vi "ObjDet_Read_Dataset_by_File_Paths_v1.1.vi"(0 "Annotation File Paths":path[](array[path]), 1 "Unique labels":string[](array[string]), 5 "Image File Paths":path[](array[path]), 7 "Img Height":i32, 9 "Img Width":i32, 11 "error in (no error)":errorcluster, 12 "Img Type":enum16{"Grayscale", "RGB"}(ring)) -> (4 "NN_DataSet(In3D_OutBBox)":T1={"Inputs Ref."=variant(refnum<data-value> refnum), "Dataset_Size"=0, "Dims_In"={"C"=0, "H"=0, "W"=0}, "Outputs Refs"=refnum, "No of Classes "=0, "Labels"=[], "File Paths"=[]}, 6 "Anchors":dbl[][](array[numeric]), 8 "Total annotations":i32, 15 "error out":errorcluster)   [LabVIEW 2020]
uses:
  <vilib>/Ngene/Deep Learning Toolkit/Toolkit/NN_Data/API/DataSet/DataSet_Types/NN_DataSet(In3D_OutBBox).ctl
  <vilib>/Ngene/Deep Learning Toolkit/Toolkit/NN_Data/API/NN_Dims(C,H,W).ctl
  <vilib>/Ngene/Deep Learning Toolkit/Toolkit/NN_Data/Controls/DataRef_Types/1D/NN_Data_ref(1D_BBox).ctl
  <vilib>/Ngene/Deep Learning Toolkit/Toolkit/NN_Data/API/Data/Detection_Types/NN_Image_Annotations.ctl
  <vilib>/Ngene/Deep Learning Toolkit/Toolkit/NN_Data/API/Data/Detection_Types/NN_BBox_Annotation.ctl
  <vilib>/Ngene/Deep Learning Toolkit/Toolkit/NN_Data/API/Data/Detection_Types/NN_BBox.ctl
  <vilib>/Ngene/Deep Learning Toolkit/Toolkit/NN_Data/API/Data/Detection_Types/NN_BBox_Format_Conversion_Direction.ctl
  <vilib>/Analysis/baseanly.llb/Mean (DBL).vi
  <vilib>/vision/NI_Vision_Development_Module.lvlib
  <vilib>/Ngene/Deep Learning Toolkit/Toolkit/Deep_Learning_Toolkit_by_Ngene.lvlib
  <vilib>/Analysis/NI_AALBase.lvlib
panel:
  out "Array":path[](array[path])
  out "Annotations with missing Imgs":path[](array[path])
  out "Img Paths with missing Annotation":path[](array[path])
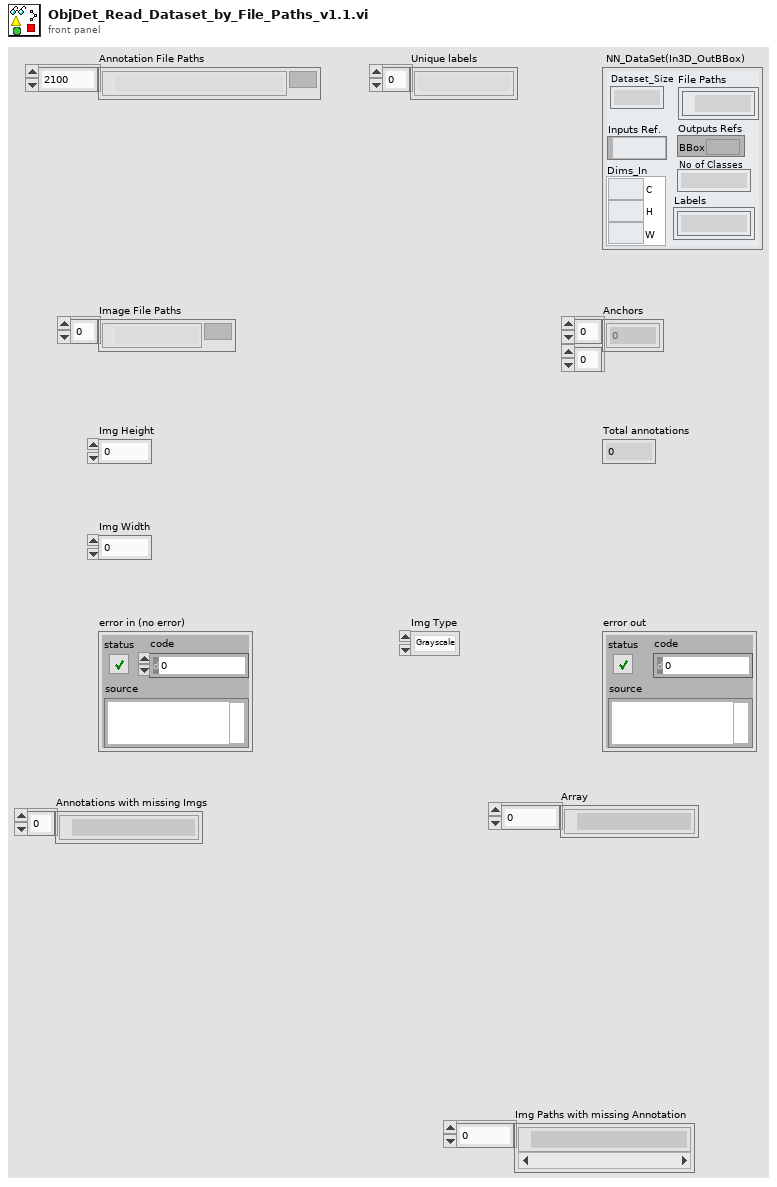
[diagram p1: front panel]
types:
  T1 = typedef "Deep_Learning_Toolkit_by_Ngene.lvlib/NN_DataSet(In3D_OutBBox).ctl" = cluster{"Inputs Ref.":variant, "Dataset_Size":i32, "Dims_In":T2, "Outputs Refs":T3, "No of Classes ":i32, "Labels":string[], "File Paths":path[]}
  T2 = typedef "Deep_Learning_Toolkit_by_Ngene.lvlib/NN_Dims(C,H,W).ctl" = cluster{"C":i32, "H":i32, "W":i32}
  T3 = typedef "Deep_Learning_Toolkit_by_Ngene.lvlib/NN_Data_ref(1D_BBox).ctl" = refnum<data-value>
  T4 = typedef "Deep_Learning_Toolkit_by_Ngene.lvlib/NN_Image_Annotations.ctl" = cluster{"Image Annotations":T5[]}
  T5 = typedef "Deep_Learning_Toolkit_by_Ngene.lvlib/NN_BBox_Annotation.ctl" = cluster{"Class":i32, "BBox":T6}
  T6 = typedef "Deep_Learning_Toolkit_by_Ngene.lvlib/NN_BBox.ctl" = cluster{"x":sgl, "y":sgl, "w":sgl, "h":sgl}
  T7 = typedef "Deep_Learning_Toolkit_by_Ngene.lvlib/NN_BBox_Format_Conversion_Direction.ctl" = enum16{"SS_to_CWH", "CWH_to_SS"}
  T8 = typedef "Image Type" = u32
  T9 = typedef "IMAQ Image.ctl" = refnum<image>
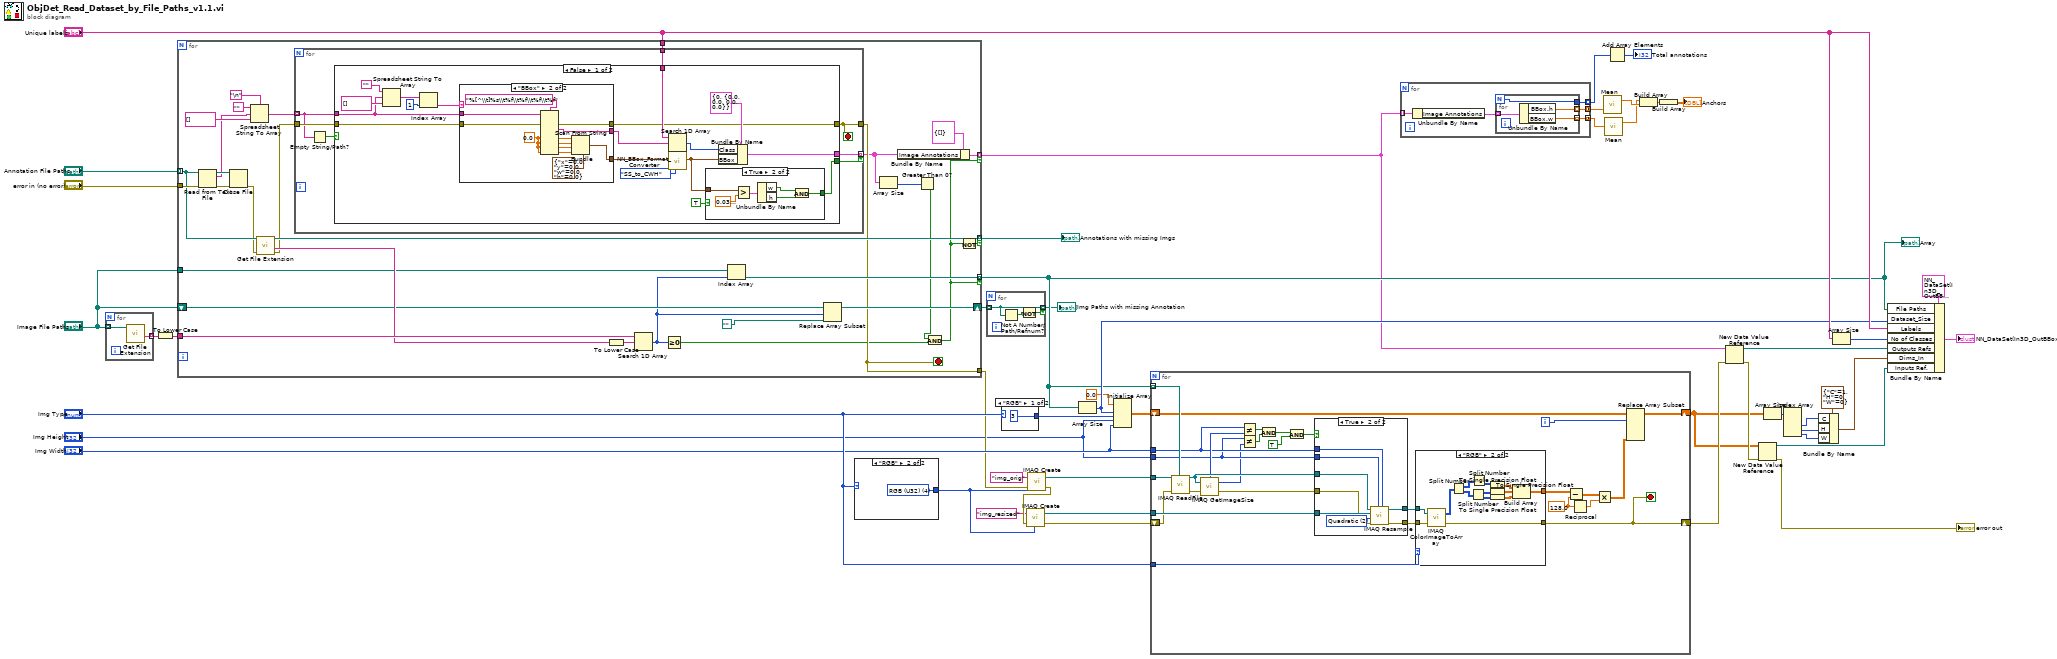
[diagram p0: block diagram]
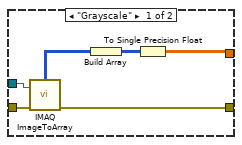
[diagram p2: hidden frame]
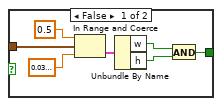
[diagram p4: hidden frame]
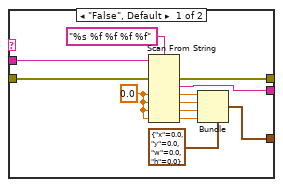
[diagram p5: hidden frame]
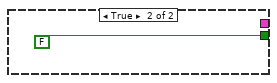
[diagram p6: hidden frame]
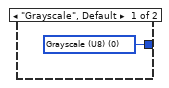
[diagram p7: hidden frame]
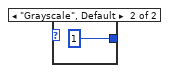
[diagram p8: hidden frame]
diagram:
  n1 = for {
    tunnel: "Image File Paths" -> [w51] mode=indexing
    tunnel: [w50] -> w14 mode=indexing
    n2 = call <vilib>:"Get File Extension.vi"("file"=w51) -> ("filename without extension"=w50:string)  [unwired: 6 in, 4 out]
  }
  n3 = To Lower Case(string=w14) -> (all lower case string=w40:string[])
  n4 = for {
    tunnel: "Annotation File Paths" -> [w61] mode=indexing
    tunnel: "Image File Paths" -> [w76]
    tunnel: [w79] -> w44 mode=indexing if=w54
    tunnel: [w78] -> w10 mode=indexing if=w54
    tunnel: "error in (no error)" -> [w69]
    tunnel: [w57] -> w27
    tunnel: w40 -> [w81]
    tunnel: [w60] -> w16 mode=indexing if=w77
    shift-right: [w75] -> w17
    shift-left: "Image File Paths" -> [w74]
    tunnel: "Unique labels" -> [w62]
    stop <- w57 stop-if-true
    n5 = Read from Text File(file (use dialog)=w61, error in=w69) -> (refnum out=w71:refnum<file>, text=w63:string, error out=w70:errorcluster)  [unwired: 2 in, 1 out]
    n6 = Close File(refnum=w71, error in=w70) -> (error out=w59:errorcluster)  [unwired: 1 out]
    n7 = Spreadsheet String To Array(delimiter (Tab)="\n", format string="", spreadsheet string=w63, array type (2D Dbl)=string[] []) -> (array=w65:string[])
    n8 = call <vilib>:"Get File Extension.vi"("error in (no error)"=w59, "file"=w61) -> ("error out"=w58:errorcluster, "filename without extension"=w80:string, "dup file"=w60:path)  [unwired: 5 in, 2 out]
    n9 = for {
      tunnel: w65 -> [w85] mode=indexing
      tunnel: w58 -> [w89]
      tunnel: [w86] -> w57
      tunnel: w62 -> [w88]
      tunnel: [w87] -> w56 mode=indexing if=w83
      stop <- w86 stop-if-true
      n10 = Empty String/Path?(string/path=w85) -> (empty?=w84:bool)
      n11 = case shown="False" w84 {
        tunnel: w89 -> [w103 _]
        tunnel: w88 -> [w101 _]
        tunnel: [w96 _] -> w87
        tunnel: [w95 _] -> w86
        tunnel: w85 -> [w93 _]
        tunnel: [w91 FALSE] -> w83
        frame False {
          n12 = Spreadsheet String To Array(format string="", spreadsheet string=w93, array type (2D Dbl)=string[] []) -> (array=w106:string[])  [unwired: 1 in]
          n13 = Index Array(array=w106, index=1) -> (element=w104:string)
          n14 = case shown="\"BBox\"" w104 {
            tunnel: w93 -> [w131 w144]
            tunnel: w103 -> [w130 w143]
            tunnel: [w129 w142] -> w95
            tunnel: [w122 w134] -> w98
            tunnel: [w121 w135] -> w102
            frame "False", Default {
              w126 = sgl 0.0 ("h")
              n15 = Scan From String(format string="%s %f %f %f %f", input string=w131, error in=w130, default 2=w126, default 3=w126, default 4=w126, default 5=w126) -> (error out=w129:errorcluster, output 1=w121:string, output 2=w127:sgl, output 3=w125:sgl, output 4=w124:sgl, output 5=w123:sgl)  [unwired: 2 in, 2 out]
              n16 = Bundle(cluster=T6 {"x"=0.0, "y"=0.0, "w"=0.0, "h"=0.0} ("Box"), "x"=w127, "y"=w125, "w"=w124, "h"=w123) -> (w122:T6)
            }
            frame "BBox" {
              w136 = sgl 0.0 ("h")
              n17 = Scan From String(format string="%[^\\t]%s\\t%f\\t%f\\t%f\\t%f", input string=w144, error in=w143, default 3=w136, default 4=w136, default 5=w136, default 6=w136) -> (error out=w142:errorcluster, output 1=w135:string, output 3=w140:sgl, output 4=w139:sgl, output 5=w138:sgl, output 6=w137:sgl)  [unwired: 4 in, 2 out]
              n18 = Bundle(cluster=T6 {"x"=0.0, "y"=0.0, "w"=0.0, "h"=0.0} ("Box"), "x"=w140, "y"=w139, "w"=w138, "h"=w137) -> (w134:T6)
            }
          }
          n19 = Search 1D Array(1D array=w101, element=w102) -> (index of element=w100:i32)  [unwired: 1 in]
          n20 = call <vilib>:"NN_BBox_Format_Converter.vi"("Conversion_Direction"=NN_BBox_Format_Conversion_Direction."SS_to_CWH" ("Format_Transform"), "BBox in"=w98) -> ("BBox out"=w92:T6)  [unwired: 9 in]
          n21 = case shown="True" TRUE {
            tunnel: w92 -> [w114 w120]
            tunnel: [w110 w117] -> w91
            frame False {
              n22 = In Range and Coerce(upper limit=sgl 0.5 ("x"), x=w114, lower limit=sgl 0.04 ("x")) -> (In Range?=w111:cluster{"x":bool, "y":bool, "w":bool, "h":bool})  [unwired: 1 out]
              n23 = Unbundle By Name(w111) -> ("w"=w109:bool, "h"=w108:bool)
              n24 = And(x=w109, y=w108) -> (x .and. y?=w110:bool)
            }
            frame True {
              n25 = Greater?(x=w120, y=sgl 0.04 ("h")) -> (0:w119:cluster{"x":bool, "y":bool, "w":bool, "h":bool})
              n26 = Unbundle By Name(w119) -> ("w"=w115:bool, "h"=w118:bool)
              n27 = And(x=w115, y=w118) -> (x .and. y?=w117:bool)
            }
          }
          n28 = Bundle By Name(cluster=T5 {"Class"=0, "BBox"={"x"=0.0, "y"=0.0, "w"=0.0, "h"=0.0}} ("BoxC"), "Class"=w100, "BBox"=w92) -> (w96:T5)
        }
        frame True {
        }
      }
    }
    n29 = To Lower Case(string=w80) -> (all lower case string=w68:string)
    n30 = Search 1D Array(1D array=w81, element=w68) -> (index of element=w73:i32)  [unwired: 1 in]
    n31 = Greater Or Equal To 0?(x=w73) -> (x >= 0?=w52:bool)
    n32 = Index Array(array=w76, index=w73) -> (element=w79:path)
    n33 = Replace Array Subset(array=w74, new element=path "" ("new element/subarray"), index=w73) -> (w75:path[])
    n34 = Array Size(array=w56) -> (size(s)=w55:i32)
    n35 = Bundle By Name(cluster=T4 {"Image Annotations"=[]} ("Image_Truths"), "Image Annotations"=w56) -> (w78:T4)
    n36 = Greater Than 0?(x=w55) -> (x > 0?=w53:bool)
    n37 = And(x=w53, y=w52) -> (x .and. y?=w54:bool)
    n38 = Not(x=w54) -> (.not. x?=w77:bool)
  }
  "Annotations with missing Imgs" <- w16
  "Array" <- w44
  n39 = case shown="\"RGB\"" "Img Type" {
    tunnel: [w146 w147] -> w34
    frame "Grayscale", Default {
      w146 = T8 0 items=["Grayscale (U8)", "Grayscale (I16)", "Grayscale (SGL)", "Complex (CSG)", "RGB (U32)", "HSL (U32)", "RGB (U64)", "Grayscale (U16)"] ("Image Type")
    }
    frame "RGB" {
      w147 = T8 4 items=["Grayscale (U8)", "Grayscale (I16)", "Grayscale (SGL)", "Complex (CSG)", "RGB (U32)", "HSL (U32)", "RGB (U64)", "Grayscale (U16)"] ("Image Type")
    }
  }
  n40 = for {
    tunnel: w17 -> [w150] mode=indexing
    tunnel: [w150] -> w22 mode=indexing if=w148
    n41 = Not A Number/Path/Refnum?(number/path/refnum=w150) -> (NaN/Path/Refnum?=w149:bool)
    n42 = Not(x=w149) -> (.not. x?=w148:bool)
  }
  "Img Paths with missing Annotation" <- w22
  n43 = case shown="\"RGB\"" "Img Type" {
    tunnel: [3 1] -> w18
    frame "RGB" {
    }
    frame "Grayscale", Default {
    }
  }
  n44 = call "IMAQ Create"("Image Name"="img_orig", "Image Type"=w34, "error in (no error)"=w27) -> ("New Image"=w12:T9, "error out"=w26:errorcluster)  [unwired: 2 in]
  n45 = call "IMAQ Create"("Image Name"="img_resized", "Image Type"=w34, "error in (no error)"=w26) -> ("New Image"=w21:T9, "error out"=w25:errorcluster)  [unwired: 2 in]
  n46 = Array Size(array=w44) -> (size(s)=w45:i32)
  n47 = Initialize Array(sgl 0.0 ("element"), w45, w18, "Img Height", "Img Width") -> (w23:sgl[][][][])
  n48 = for {
    tunnel: w12 -> [w180]
    tunnel: w21 -> [w178]
    tunnel: w44 -> [w176] mode=indexing
    shift-right: [w174] -> w5
    shift-left: w23 -> [w175]
    tunnel: "Img Height" -> [w166]
    tunnel: "Img Width" -> [w167]
    shift-right: [w161] -> w32
    shift-left: w25 -> [w172]
    tunnel: "Img Type" -> [w160]
    i -> [w173]
    stop <- w161 stop-if-true
    w156 = sgl 128.0 ("element")
    n49 = call "IMAQ ReadFile"("File Path"=w176, "error in (no error)"=w172, "Image"=w180) -> ("error out"=w171:errorcluster, "Image Out"=w169:T9)  [unwired: 4 in, 3 out]
    n50 = call "IMAQ GetImageSize"("Image"=w169, "error in (no error)"=w171) -> ("Y Resolution"=w165:i32, "X Resolution"=w168:i32, "error out"=w170:errorcluster)  [unwired: 2 in]
    n51 = Not Equal?(x=w167, y=w168) -> (x != y?=w164:bool)
    n52 = Not Equal?(x=w166, y=w165) -> (x != y?=w163:bool)
    n53 = Compound Arithmetic op=AND(w164, w163) -> (w162:bool)
    n54 = And(x=w162, y=TRUE ("value")) -> (x .and. y?=w159:bool)
    n55 = case shown="True" w159 {
      tunnel: w169 -> [w201 w209]
      tunnel: [w201 w208] -> w179
      tunnel: w178 -> [_ w207]
      tunnel: w170 -> [w200 w206]
      tunnel: [w200 w205] -> w177
      tunnel: w166 -> [_ w204]
      tunnel: w167 -> [_ w203]
      frame False {
      }
      frame True {
        w202 = u32 2 items=["Zero Order", "Bi-Linear", "Quadratic", "Cubic Spline"] ("Interpolation Type")
        n56 = call "IMAQ Resample"("X Resolution"=w203, "Y Resolution"=w204, "error in (no error)"=w206, "Interpolation Type"=w202, "Image Dst"=w207, "Image Src"=w209) -> ("error out"=w205:errorcluster, "Image Dst Out"=w208:T9)  [unwired: 4 in]
      }
    }
    n57 = case shown="\"RGB\"" w160 {
      tunnel: w179 -> [w186 w199]
      tunnel: w177 -> [w185 w198]
      tunnel: [w183 w196] -> w161
      tunnel: [w181 w187] -> w155
      frame "Grayscale" {
        n58 = call "IMAQ ImageToArray"("error in (no error)"=w185, "Image"=w186) -> ("error out"=w183:errorcluster, "Image Pixels (U8)"=w184:u8[][])  [unwired: 2 in, 3 out]
        n59 = Build Array(w184) -> (w182:u8[][][])
        n60 = To Single Precision Float(number=w182) -> (single precision float=w181:sgl[][][])
      }
      frame "RGB" {
        n61 = call "IMAQ ColorImageToArray"("Image"=w199, "error in (no error)"=w198) -> ("Image Pixels (U32)"=w197:u32[][], "error out"=w196:errorcluster)  [unwired: 2 in, 1 out]
        n62 = Split Number(x=w197) -> (hi(x)=w194:u16[][], lo(x)=w195:u16[][])
        n63 = Split Number(x=w195) -> (hi(x)=w192:u8[][], lo(x)=w191:u8[][])
        n64 = Split Number(x=w194) -> (lo(x)=w193:u8[][])  [unwired: 1 out]
        n65 = To Single Precision Float(number=w193) -> (single precision float=w190:sgl[][])
        n66 = To Single Precision Float(number=w192) -> (single precision float=w189:sgl[][])
        n67 = To Single Precision Float(number=w191) -> (single precision float=w188:sgl[][])
        n68 = Build Array(w190, w189, w188) -> (w187:sgl[][][])
      }
    }
    n69 = Subtract(x=w155, y=w156) -> (x-y=w157:sgl[][][])
    n70 = Reciprocal(x=w156) -> (1/x=w153:sgl)
    n71 = Multiply(x=w157, y=w153) -> (x*y=w154:sgl[][][])
    n72 = Replace Array Subset(array=w175, new element=w154, index (dim 0)=w173) -> (w174:sgl[][][][])  [unwired: 3 in]
  }
  n73 = for {
    tunnel: w10 -> [w214] mode=indexing
    tunnel: [w212] -> w4 mode=concatenating
    tunnel: [w211] -> w3 mode=concatenating
    tunnel: [w210] -> w2 mode=indexing
    n74 = Unbundle By Name(w214) -> ("Image Annotations"=w213:T5[])
    n75 = for {
      N -> [w215]
      tunnel: w213 -> [w218] mode=indexing
      tunnel: [w217] -> w212 mode=indexing
      tunnel: [w216] -> w211 mode=indexing
      tunnel: [w215] -> w210
      n76 = Unbundle By Name(w218) -> ("BBox.h"=w217:sgl, "BBox.w"=w216:sgl)
    }
  }
  n77 = call-poly <vilib>:"Mean.vi"("X"=w4) -> ("mean"=w9:dbl)  [unwired: 1 out]
  n78 = call-poly <vilib>:"Mean.vi"("X"=w3) -> ("mean"=w8:dbl)  [unwired: 1 out]
  n79 = Add Array Elements(numeric array=w2) -> (sum=→"Total annotations":i32)
  n80 = Build Array(w8, w9) -> (w7:dbl[])
  n81 = Build Array(w7) -> (→"Anchors":dbl[][])
  n82 = New Data Value Reference(data value=w10, error in=w32) -> (data value reference=w31:refnum<data-value>, error out=w33:errorcluster)
  n83 = New Data Value Reference(data value=w5, error in=w33) -> (data value reference=w30:refnum<data-value>, error out=→"error out":errorcluster)
  n84 = Array Size(array=w5) -> (size(s)=w36:i32[])
  n85 = Index Array(array=w36) -> (element #2=w37:i32, element #3=w38:i32, element #4=w39:i32)  [unwired: 4 in, 1 out]
  n86 = Bundle By Name(cluster=T2 {"C"=1, "H"=0, "W"=0} ("Dims"), "C"=w37, "H"=w38, "W"=w39) -> (w43:T2)
  n87 = Array Size(array="Unique labels") -> (size(s)=w42:i32)
  n88 = Bundle By Name(cluster=T1 {"Inputs Ref."=variant(refnum<data-value> refnum), "Dataset_Size"=0, "Dims_In"={"C"=0, "H"=0, "W"=0}, "Outputs Refs"=refnum, "No of Classes "=0, "Labels"=["large", "small"], "File Paths"=[]} ("Train DataSet"), "File Paths"=w44, "Dataset_Size"=w45, "Labels"="Unique labels", "No of Classes"=w42, "Outputs Refs"=w31, "Dims_In"=w43, "Inputs Ref."=w30) -> (→"NN_DataSet(In3D_OutBBox)":T1)
